vi "Periodic Tasks.vi"(8 "error in":errorcluster) -> ()   [LabVIEW 2013]
doc: "This VI runs in parallel to other tasks. It can contain as many user-defined periodic loops as you need. These can carry out PID or other sorts of timed response."
uses:
  <vilib>/Rock Robotics/SystemInterfaces/Utilities/FPGA_UtilitiesLED Source.ctl
  <vilib>/Rock Robotics/SystemInterfaces/Utilities/FPGA_UtilitiesLED State.ctl
  Robot Global Data.vi
  <vilib>/Rock Robotics/WPI/Compressor/WPI_CompressorGetSetRefNum.vi
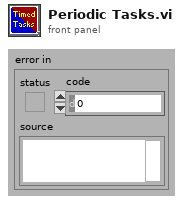
[diagram p1: front panel]
types:
  T1 = typedef "WPI_DigitalInputDevRef.ctl" = cluster{"DevStatus":errorcluster, "DIO Channel":T2, "Digital Module":T3}
  T2 = typedef "FPGA_DIOChannel.ctl" = enum8{"DIO 1", "DIO 2", "DIO 3", "DIO 4", "DIO 5", "DIO 6", "DIO 7", "DIO 8", "DIO 9", "DIO 10", "DIO 11", "DIO 12", "DIO 13", "DIO 14", "Invalid"}
  T3 = typedef "FPGA_TypedefDigitalModule.ctl" = enum16{"Digital Module 1", "Digital Module 2"}
  T4 = cluster{"DigitalInputDevRef":T1, "DigitalInputDevRef":T1}
  T5 = typedef "WPI_GyroDevRef.ctl" = cluster{"DevStatus":errorcluster, "Analog Module":T6, "Analog Channel":T7, "Offset":dbl, "Gain (VoltsPerDegree/Second)":dbl}
  T6 = typedef "FPGA_TypedefAnalogModule.ctl" = enum16{"Analog Module 1", "Analog Module 2"}
  T7 = typedef "FPGA_AIChannel.ctl" = enum8{"AI 1", "AI 2", "AI 3", "AI 4", "AI 5", "AI 6", "AI 7", "AI 8", "Invalid"}
  T8 = typedef "FPGA_UtilitiesLED State.ctl" = enum16{"Off", "On", "Toggle"}
  T9 = typedef "FPGA_UtilitiesLED Source.ctl" = enum16{"User LED", "FPGA LED"}
  T10 = typedef "WPI_CompressorDevRef.ctl" = cluster{"DevStatus":errorcluster, "DigitalInputDevRef":T1, "RelayDevRef":T11}
  T11 = typedef "WPI_RelayDevRef.ctl" = cluster{"DevStatus":errorcluster, "Relay Channel":T12, "Digital Module":T3, "Relay Direction":T13}
  T12 = typedef "FPGA_DIORelayChannel.ctl" = enum8{"Relay 1", "Relay 2", "Relay 3", "Relay 4", "Relay 5", "Relay 6", "Relay 7", "Relay 8", "Invalid"}
  T13 = typedef "WPI_RelayDirection.ctl" = enum16{"Both directions", "Forward only", "Reverse only"}
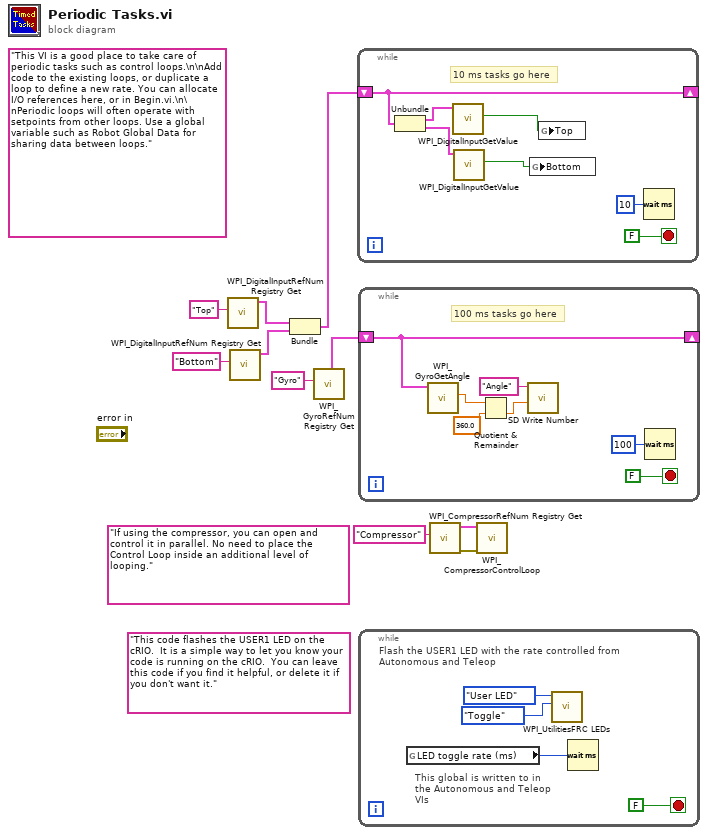
[diagram p0: block diagram]
diagram:
  (unwired) "If using the compressor, you can open and control it in parallel. No need to place the Control Loop inside an additional level of looping."
  (unwired) "This code flashes the USER1 LED on the cRIO.  It is a simple way to let you know your code is running on the cRIO.  You can leave this code if you find it helpful, or delete it if you don't want it."
  (unwired) "This VI is a good place to take care of periodic tasks such as control loops.\n\nAdd code to the existing loops, or duplicate a loop to define a new rate. You can allocate I/O references here, or in Begin.vi.\n\nPeriodic loops will often operate with setpoints from other loops. Use a global variable such as Robot Global Data for sharing data between loops."
  n1 = call <vilib>:"WPI_DigitalInputRefNum Registry Get.vi"("refnum name"="Top") -> ("DigitalInputDevRef"=w5:T1)  [unwired: 9 in, 1 out]
  n2 = call <vilib>:"WPI_DigitalInputRefNum Registry Get.vi"("refnum name"="Bottom") -> ("DigitalInputDevRef"=w4:T1)  [unwired: 9 in, 1 out]
  n3 = Bundle("DigitalInputDevRef"=w5, "DigitalInputDevRef"=w4) -> (w3:T4)  [unwired: 1 in]
  n4 = call <vilib>:"WPI_GyroRefNum Registry Get.vi"("refnum name"="Gyro") -> ("GyroDevRef"=w1:T5)  [unwired: 9 in, 1 out]
  n5 = while {
    shift-right: [w15] -> _
    shift-left: w3 -> [w15]
    stop <- FALSE stop-if-true
    # "10 ms tasks go here"
    n6 = Unbundle(w15) -> ("DigitalInputDevRef"=w14:T1, "DigitalInputDevRef"=w13:T1)
    n7 = call <vilib>:"WPI_DigitalInputGetValue.vi"("DigitalInputDevRef"=w14) -> ("Value"=w12:bool)  [unwired: 8 in, 2 out]
    n8 = call <vilib>:"WPI_DigitalInputGetValue.vi"("DigitalInputDevRef"=w13) -> ("Value"=w11:bool)  [unwired: 8 in, 2 out]
    n9 = global write "Robot Global Data.vi" "Bottom"(w11) -> ()
    n10 = global write "Robot Global Data.vi" "Top"(w12) -> ()
    n11 = Wait (ms)(milliseconds to wait=u32 10) -> ()  [unwired: 1 out]
  }
  n12 = while {
    shift-right: [w22] -> _
    shift-left: w1 -> [w22]
    stop <- FALSE stop-if-true
    # "100 ms tasks go here"
    n13 = call <vilib>:"WPI_GyroGetAngle.vi"("GyroDevRef"=w22) -> ("Angle"=w21:dbl)  [unwired: 7 in, 3 out]
    n14 = Quotient & Remainder(x=w21, y=360.0) -> (floor(x/y)=w20:dbl)  [unwired: 1 out]
    n15 = call <vilib>:"SD Write Number.vi"("Numeric"=w20, "Name"="Angle") -> ()  [unwired: 8 in, 2 out]
    n16 = Wait (ms)(milliseconds to wait=u32 100) -> ()  [unwired: 1 out]
  }
  n17 = while {
    stop <- FALSE stop-if-true
    # "This global is written to in the Autonomous and Teleop VIs"
    # "Flash the USER1 LED with the rate controlled from Autonomous and Teleop"
    n18 = global read "Robot Global Data.vi" "LED toggle rate (ms)"() -> (w25:u32)
    n19 = call <vilib>:"WPI_UtilitiesFRC LEDs.vi"("State"=FPGA_UtilitiesLED_State."Toggle", "LED Type"=FPGA_UtilitiesLED_Source."User LED") -> ()  [unwired: 1 in, 9 out]
    n20 = Wait (ms)(milliseconds to wait=w25) -> ()  [unwired: 1 out]
  }
  n21 = call <vilib>:"WPI_CompressorRefNum Registry Get.vi"("refnum name"="Compressor") -> ("error out"=w9:errorcluster, "CompressorDevRef"=w8:T10)  [unwired: 9 in]
  n22 = call <vilib>:"WPI_CompressorControlLoop.vi"("error in (no error)"=w9, "CompressorDevRef"=w8) -> ()  [unwired: 10 in]
